vi "Cluster textbool name.vi"(8 "error in (no error)":errorcluster, 10 "Station Name":string[](array[string]), 11 "Clust Refnum":refnum<vi>) -> (0 "error out":errorcluster)   [LabVIEW 2014]
uses:
  Type'def/Shield Ctr.ctl
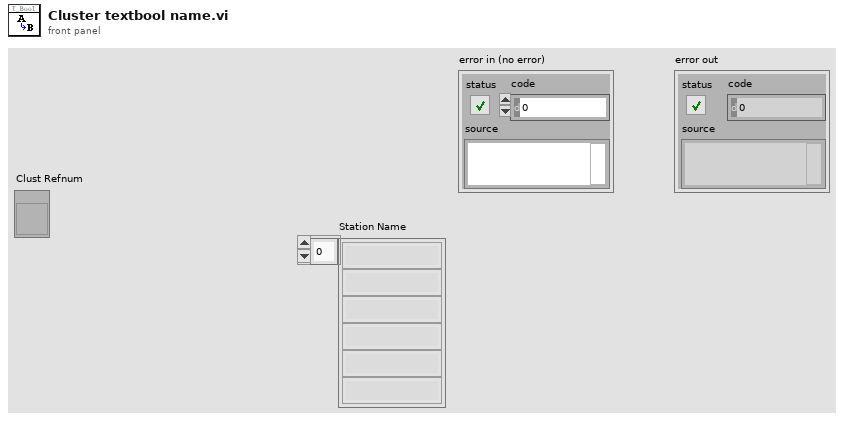
[diagram p1: front panel]
types:
  T1 = typedef "Shield Ctr.ctl" = cluster{"No.1":bool, "No.2":bool, "No.3":bool, "No.4":bool, "No.5":bool, "No.6":bool, "No.7":bool, "No.8":bool, "No.9":bool, "No.10":bool, "No.10 2":bool, "No.11":bool, "No.12":bool, "No.11 2":bool, "No.12 2":bool, "No.12 3":bool}
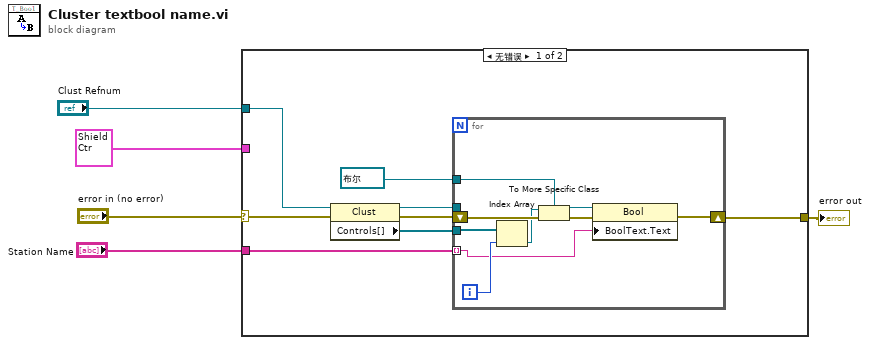
[diagram p0: block diagram]
diagram:
  n1 = case shown="无错误" "error in (no error)" {
    selector: "error in (no error)" -> [w13 w23]
    tunnel: "Clust Refnum" -> [w12 _]
    tunnel: T1 {"No.1"=FALSE, "No.2"=FALSE, "No.3"=FALSE, "No.4"=FALSE, "No.5"=FALSE, "No.6"=FALSE, "No.7"=FALSE, "No.8"=FALSE, "No.9"=FALSE, "No.10"=FALSE, "No.10 2"=FALSE, "No.11"=FALSE, "No.12"=FALSE, "No.11 2"=FALSE, "No.12 2"=FALSE, "No.12 3"=FALSE} ("Shield") -> [_ _]
    tunnel: "Station Name" -> [w11 _]
    tunnel: [w7 w23] -> w2
    frame No Error {
      n2 = property class="Clust"(reference=w12, error in=w13) -> (reference out=w8:refnum<vi>, error out=w9:errorcluster, "Controls[]"=w10:refnum<vi>[])
      n3 = for {
        tunnel: w11 -> [w14] mode=indexing
        tunnel: w10 -> [w22]
        tunnel: w8 -> [_]
        shift-right: [w20] -> w7
        shift-left: w9 -> [w19]
        tunnel: refnum<vi> refnum ("Bool Refnum") -> [w15]
        i -> [w21]
        n4 = Index Array(array=w22, index=w21) -> (element=w18:refnum<vi>)
        n5 = To More Specific Class(target class=w15, reference=w18, error in=w19) -> (specific class reference=w16:refnum<vi>, error out=w17:errorcluster)
        n6 = property class="Bool"(reference=w16, error in=w17, "BoolText.Text"=w14) -> (error out=w20:errorcluster)  [unwired: 1 out]
      }
    }
    frame Error {
    }
  }
  "error out" <- w2
